vi "GetTaskChecked.vi"(8 "error in (no error)":errorcluster, 11 "TaskList in":refnum<class "TaskList.lvclass">) -> (0 "error out":errorcluster, 2 "TaskChecked":bool[](array[boolean]), 3 "TaskList out":refnum<class "TaskList.lvclass">)   [LabVIEW 2021, in "LvMarkdown.lvlib" / "TaskList.lvclass"]
uses:
  TaskList.lvclass
  TaskList.lvclass/TaskList.ctl
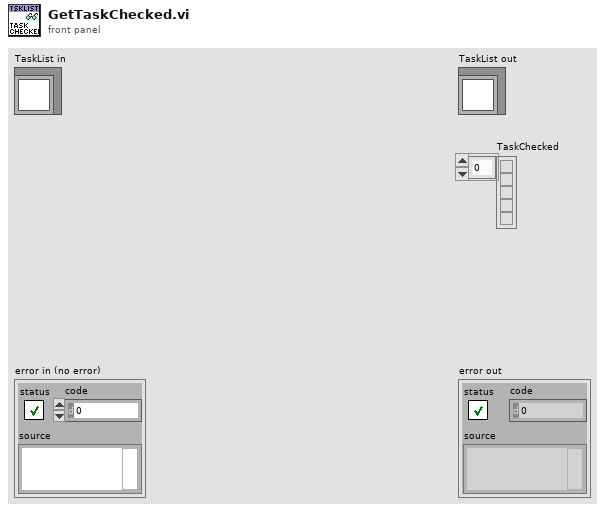
[diagram p1: front panel]
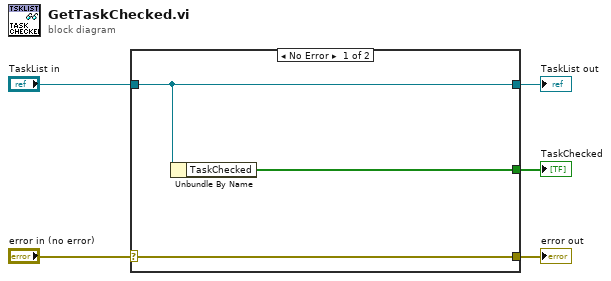
[diagram p0: block diagram]
diagram:
  n1 = case shown="No Error" "error in (no error)" {
    selector: "error in (no error)" -> [w8 w9]
    tunnel: [w8 w9] -> w4
    tunnel: [w7 w10] -> w2
    tunnel: "TaskList in" -> [w7 w10]
    tunnel: [w6 _] -> w1
    frame No Error {
      n2 = Unbundle By Name(w7) -> ("TaskChecked"=w6:bool[])
    }
    frame Error {
    }
  }
  "error out" <- w4
  "TaskList out" <- w2
  "TaskChecked" <- w1
